vi "celtic chant music sub vi.vi"(11 "BrickReference in":T1) -> (3 "BrickReference out":T1)   [LabVIEW 2016]
uses:
  <vilib>/NXT/Subs/LVHSConnector.ctl
  <vilib>/NXT/LegoClasses/BrickReference/BrickReference.lvclass
  <vilib>/NXT/Dual Mode Library/Sound/PlayF.vi
  <vilib>/NXT/Dual Mode Library/Sound/PlayDsharp.vi
  <vilib>/NXT/Dual Mode Library/Sound/PlayC.vi
  <vilib>/NXT/Dual Mode Library/Waits/Wait_Num(msec).vi
  <vilib>/NXT/Dual Mode Library/Sound/PlayGsharp.vi
  <vilib>/NXT/Dual Mode Library/Sound/PlayG.vi
  <vilib>/NXT/Dual Mode Library/Sound/PlayE.vi
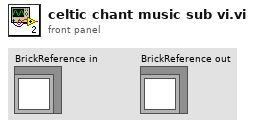
[diagram p1: front panel]
types:
  T1 = typedef "LVHSConnector.ctl" = refnum<class "BrickReference.lvclass">
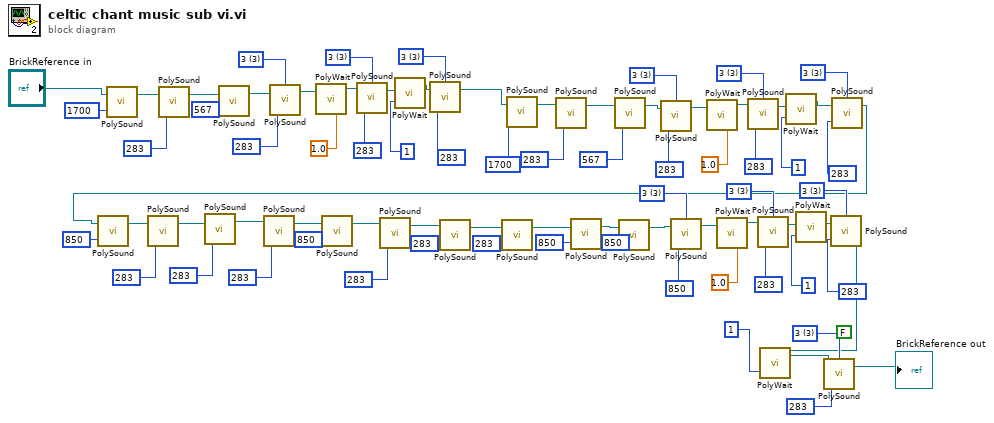
[diagram p0: block diagram]
diagram:
  w73 = u16 3 items=["3"=3, "4"=4, "5"=5, "6"=6, "7"=7] ("Octave")
  w68 = u16 3 items=["3"=3, "4"=4, "5"=5, "6"=6, "7"=7] ("Octave")
  w67 = u16 3 items=["3"=3, "4"=4, "5"=5, "6"=6, "7"=7] ("Octave")
  w66 = u16 3 items=["3"=3, "4"=4, "5"=5, "6"=6, "7"=7] ("Octave")
  w65 = u16 3 items=["3"=3, "4"=4, "5"=5, "6"=6, "7"=7] ("Octave")
  w64 = u16 3 items=["3"=3, "4"=4, "5"=5, "6"=6, "7"=7] ("Octave")
  w63 = u16 3 items=["3"=3, "4"=4, "5"=5, "6"=6, "7"=7] ("Octave")
  w62 = u16 3 items=["3"=3, "4"=4, "5"=5, "6"=6, "7"=7] ("Octave")
  w61 = u16 3 items=["3"=3, "4"=4, "5"=5, "6"=6, "7"=7] ("Octave")
  w60 = u16 3 items=["3"=3, "4"=4, "5"=5, "6"=6, "7"=7] ("Octave")
  (unwired) FALSE
  n1 = call-poly <vilib>:"PolySound.vi"("Duration (500 ms)"=u16 1700, "NXT/EV3"="BrickReference in") -> ("NXT/EV3"=w2:T1)  [unwired: 2 in]
  n2 = call-poly <vilib>:"PolySound.vi"("Duration (500 ms)"=u16 283, "NXT/EV3"=w2) -> ("NXT/EV3"=w3:T1)  [unwired: 2 in]
  n3 = call-poly <vilib>:"PolySound.vi"("Duration (500 ms)"=u16 567, "NXT/EV3"=w3) -> ("NXT/EV3"=w30:T1)  [unwired: 2 in]
  n4 = call-poly <vilib>:"PolySound.vi"("Duration (500 ms)"=u16 283, "NXT/EV3"=w30, "Octave"=w60) -> ("NXT/EV3"=w36:T1)  [unwired: 1 in]
  n5 = call-poly <vilib>:"PolyWait.vi"("Time (100 msec)"=sgl 1.0 ("Time (1 sec)"), "NXT/EV3"=w36) -> ("NXT/EV3"=w37:T1)  [unwired: 2 in]
  n6 = call-poly <vilib>:"PolySound.vi"("Duration (500 ms)"=u16 283, "NXT/EV3"=w37, "Octave"=w61) -> ("NXT/EV3"=w38:T1)  [unwired: 1 in]
  n7 = call-poly <vilib>:"PolyWait.vi"("Time (100 msec)"=u32 1, "NXT/EV3"=w38) -> ("NXT/EV3"=w39:T1)  [unwired: 2 in]
  n8 = call-poly <vilib>:"PolySound.vi"("Duration (500 ms)"=u16 283, "NXT/EV3"=w39, "Octave"=w62) -> ("NXT/EV3"=w33:T1)  [unwired: 1 in]
  n9 = call-poly <vilib>:"PolySound.vi"("Duration (500 ms)"=u16 1700, "NXT/EV3"=w33) -> ("NXT/EV3"=w7:T1)  [unwired: 2 in]
  n10 = call-poly <vilib>:"PolySound.vi"("Duration (500 ms)"=u16 283, "NXT/EV3"=w7) -> ("NXT/EV3"=w8:T1)  [unwired: 2 in]
  n11 = call-poly <vilib>:"PolySound.vi"("Duration (500 ms)"=u16 567, "NXT/EV3"=w8) -> ("NXT/EV3"=w49:T1)  [unwired: 2 in]
  n12 = call-poly <vilib>:"PolySound.vi"("Duration (500 ms)"=u16 283, "NXT/EV3"=w49, "Octave"=w63) -> ("NXT/EV3"=w44:T1)  [unwired: 1 in]
  n13 = call-poly <vilib>:"PolyWait.vi"("Time (100 msec)"=sgl 1.0 ("Time (1 sec)"), "NXT/EV3"=w44) -> ("NXT/EV3"=w45:T1)  [unwired: 2 in]
  n14 = call-poly <vilib>:"PolySound.vi"("Duration (500 ms)"=u16 283, "NXT/EV3"=w45, "Octave"=w64) -> ("NXT/EV3"=w46:T1)  [unwired: 1 in]
  n15 = call-poly <vilib>:"PolyWait.vi"("Time (100 msec)"=u32 1, "NXT/EV3"=w46) -> ("NXT/EV3"=w47:T1)  [unwired: 2 in]
  n16 = call-poly <vilib>:"PolySound.vi"("Duration (500 ms)"=u16 283, "NXT/EV3"=w47, "Octave"=w65) -> ("NXT/EV3"=w50:T1)  [unwired: 1 in]
  n17 = call-poly <vilib>:"PolySound.vi"("Duration (500 ms)"=u16 850, "NXT/EV3"=w50) -> ("NXT/EV3"=w12:T1)  [unwired: 2 in]
  n18 = call-poly <vilib>:"PolySound.vi"("Duration (500 ms)"=u16 283, "NXT/EV3"=w12) -> ("NXT/EV3"=w13:T1)  [unwired: 2 in]
  n19 = call-poly <vilib>:"PolySound.vi"("Duration (500 ms)"=u16 283, "NXT/EV3"=w13) -> ("NXT/EV3"=w17:T1)  [unwired: 2 in]
  n20 = call-poly <vilib>:"PolySound.vi"("Duration (500 ms)"=u16 283, "NXT/EV3"=w17) -> ("NXT/EV3"=w18:T1)  [unwired: 2 in]
  n21 = call-poly <vilib>:"PolySound.vi"("Duration (500 ms)"=u16 850, "NXT/EV3"=w18) -> ("NXT/EV3"=w14:T1)  [unwired: 2 in]
  n22 = call-poly <vilib>:"PolySound.vi"("Duration (500 ms)"=u16 283, "NXT/EV3"=w14) -> ("NXT/EV3"=w15:T1)  [unwired: 2 in]
  n23 = call-poly <vilib>:"PolySound.vi"("Duration (500 ms)"=u16 283, "NXT/EV3"=w15) -> ("NXT/EV3"=w19:T1)  [unwired: 2 in]
  n24 = call-poly <vilib>:"PolySound.vi"("Duration (500 ms)"=u16 283, "NXT/EV3"=w19) -> ("NXT/EV3"=w20:T1)  [unwired: 2 in]
  n25 = call-poly <vilib>:"PolySound.vi"("Duration (500 ms)"=u16 850, "NXT/EV3"=w20) -> ("NXT/EV3"=w16:T1)  [unwired: 2 in]
  n26 = call-poly <vilib>:"PolySound.vi"("Duration (500 ms)"=u16 850, "NXT/EV3"=w16) -> ("NXT/EV3"=w58:T1)  [unwired: 2 in]
  n27 = call-poly <vilib>:"PolySound.vi"("Duration (500 ms)"=u16 850, "NXT/EV3"=w58, "Octave"=w66) -> ("NXT/EV3"=w54:T1)  [unwired: 1 in]
  n28 = call-poly <vilib>:"PolyWait.vi"("Time (100 msec)"=sgl 1.0 ("Time (1 sec)"), "NXT/EV3"=w54) -> ("NXT/EV3"=w55:T1)  [unwired: 2 in]
  n29 = call-poly <vilib>:"PolySound.vi"("Duration (500 ms)"=u16 283, "NXT/EV3"=w55, "Octave"=w67) -> ("NXT/EV3"=w56:T1)  [unwired: 1 in]
  n30 = call-poly <vilib>:"PolyWait.vi"("Time (100 msec)"=u32 1, "NXT/EV3"=w56) -> ("NXT/EV3"=w70:T1)  [unwired: 2 in]
  n31 = call-poly <vilib>:"PolySound.vi"("Duration (500 ms)"=u16 283, "NXT/EV3"=w70, "Octave"=w68) -> ("NXT/EV3"=w72:T1)  [unwired: 1 in]
  n32 = call-poly <vilib>:"PolyWait.vi"("Time (100 msec)"=u32 1, "NXT/EV3"=w72) -> ("NXT/EV3"=w74:T1)  [unwired: 2 in]
  n33 = call-poly <vilib>:"PolySound.vi"("Duration (500 ms)"=u16 283, "NXT/EV3"=w74, "Octave"=w73) -> ("NXT/EV3"=→"BrickReference out":T1)  [unwired: 1 in]
